vi "RemoveBus.vi"(7 "Remove All? (F)":bool, 8 "ErrorArray In":errorcluster[](array[cluster]), 10 "clFrontPanelControlRefs":T1) -> (0 "ErrorArray Out":errorcluster[](array[cluster]))   [LabVIEW 2014, in "Bus.lvlib" / "NISTBus.lvclass"]
uses:
  NISTBus.lvclass
  Framework/FrontPanel/TypeDefs/clFrontPanelControlRefs.ctl
  FGenPlugins/MyPluginBaseClass/TypeDef/PluginParams.ctl
  WfrmGenerator/WfrmPlugins/EventPluginBaseClass/TypeDefs/dblEvtSignalArray.ctl
  FGenPlugins/MyPluginBaseClass/TypeDef/CreateArbWfrmParams.ctl
  WfrmGenerator/WfrmPlugins/EventPluginBaseClass/TypeDefs/clEvtConfig.ctl
  WfrmGenerator/WfrmModule/PublicAPI/Arguments/Requests/dblEvtParams.ctl
  FGenPlugins/MyPluginBaseClass/TypeDef/ConfigArbWfrmParams.ctl
  FGenPlugins/MyPluginBaseClass/TypeDef/TriggerParams.ctl
  <userlib>/NIST/ModuleAdminLib/ModuleAdmin/ModuleAdmin.lvclass
  <vilib>/Utility/error.llb/Error Cluster From Error Code.vi
  <vilib>/ErrorRing/Error Ring.xnode
  <userlib>/NIST/NISTErrorLib/NISTErrorLib.lvlib
  FGenModule/FGenModule.lvlib
  WfrmGenerator/WfrmModule/WfrmModule.lvlib
  Framework/TestFramework.lvlib
  Bus.lvlib
  FGenPlugins/MyPluginBaseClass/NISTFGenPluginsBase.lvclass
  WfrmGenerator/WfrmPlugins/EventPluginBaseClass/BaseWfrmPlugin.lvclass
panel:
  # "When you add a control \non the front panel, add a\nreference for it in this\ntype def.  This cluster\nwill hold all of the refer-\nences to the front panel\ncontrols in order to pass\nthese control references \nto subvis."
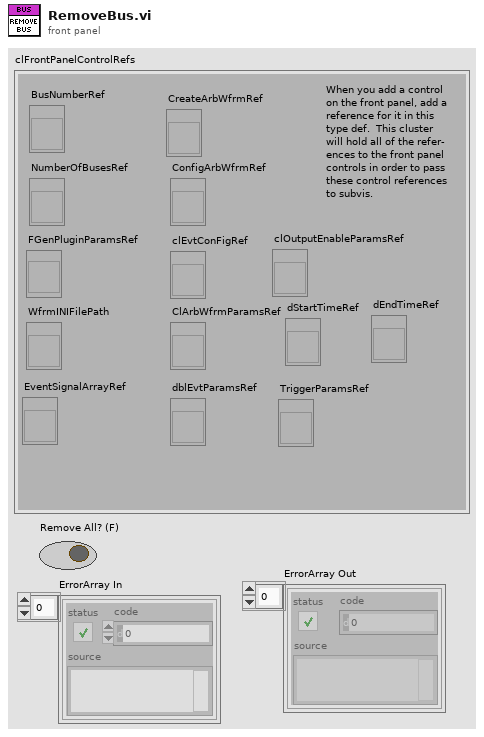
[diagram p1: front panel]
types:
  T1 = typedef "TestFramework.lvlib/clFrontPanelControlRefs.ctl" = cluster{"BusNumberRef":refnum<vi>, "NumberOfBusesRef":refnum<vi>, "FGenPluginParamsRef":refnum<vi>, "WfrmINIFilePath":refnum<vi>, "EventSignalArrayRef":refnum<vi>, "CreateArbWfrmRef":refnum<vi>, "clEvtConFigRef":refnum<vi>, "dblEvtParamsRef":refnum<vi>, "clOutputEnableParamsRef":refnum<vi>, "ConfigArbWfrmRef":refnum<vi>, "ClArbWfrmParamsRef":refnum<vi>, "dStartTimeRef":refnum<vi>, "dEndTimeRef":refnum<vi>, "TriggerParamsRef":refnum<vi>}
  T2 = typedef "TestFramework.lvlib/clFrameworkData.ctl" = cluster{"NISTBusClassInstances":refnum<class "NISTBus.lvclass">[], "NISTFGenINIFilePaths":path[], "NISTWfrmINIFilePaths":path[]}
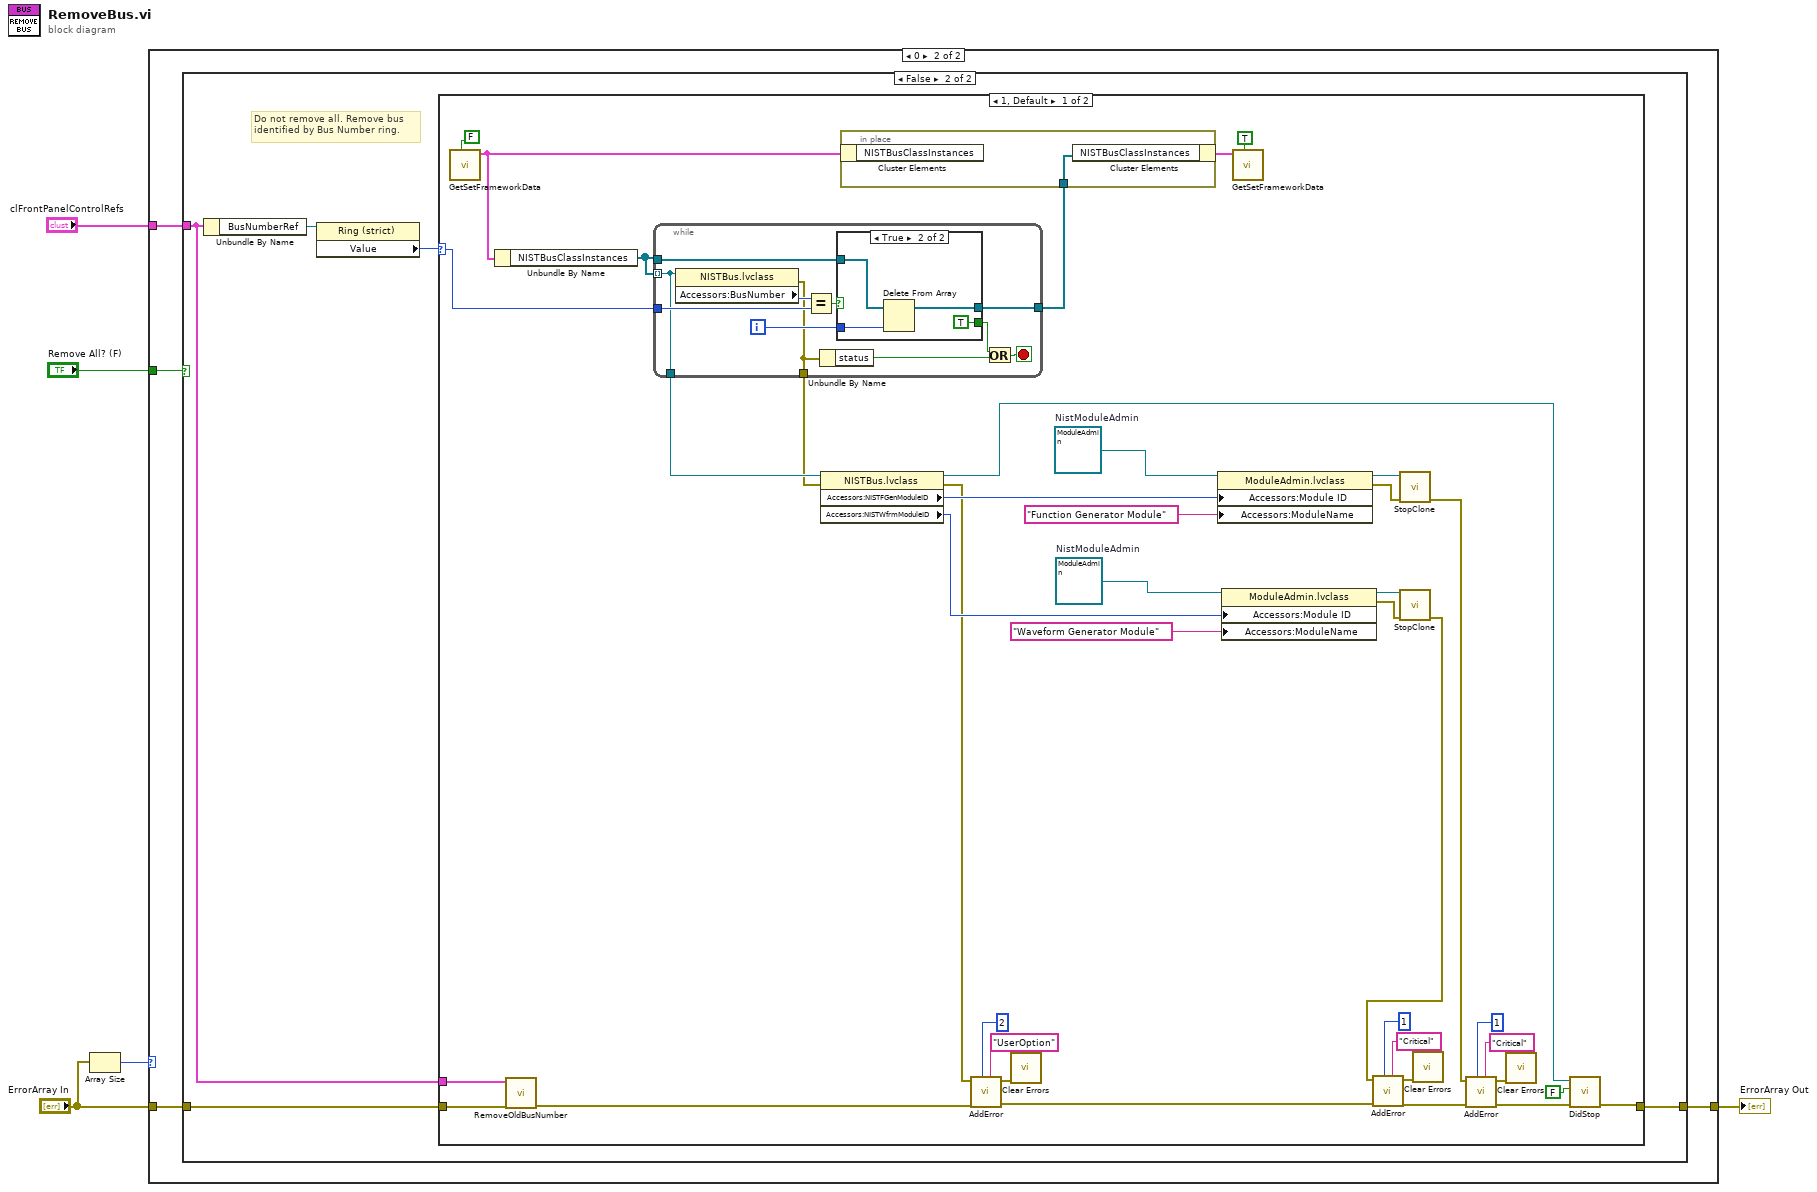
[diagram p0: block diagram]
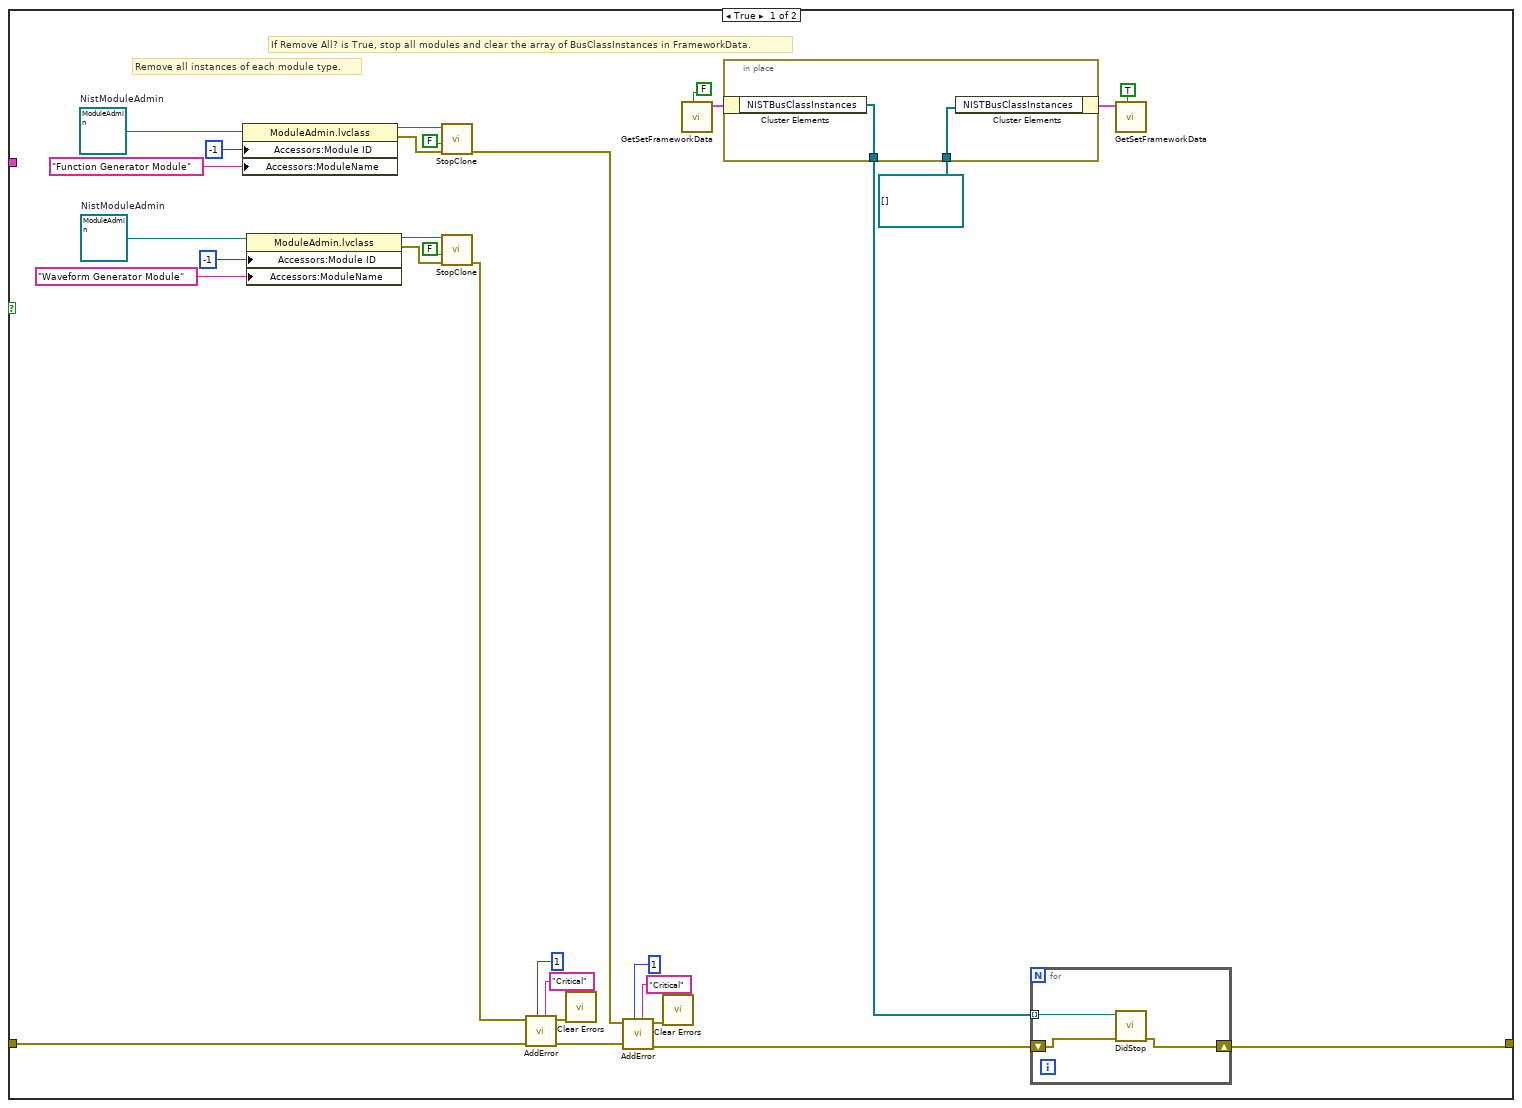
[diagram p3: hidden frame]
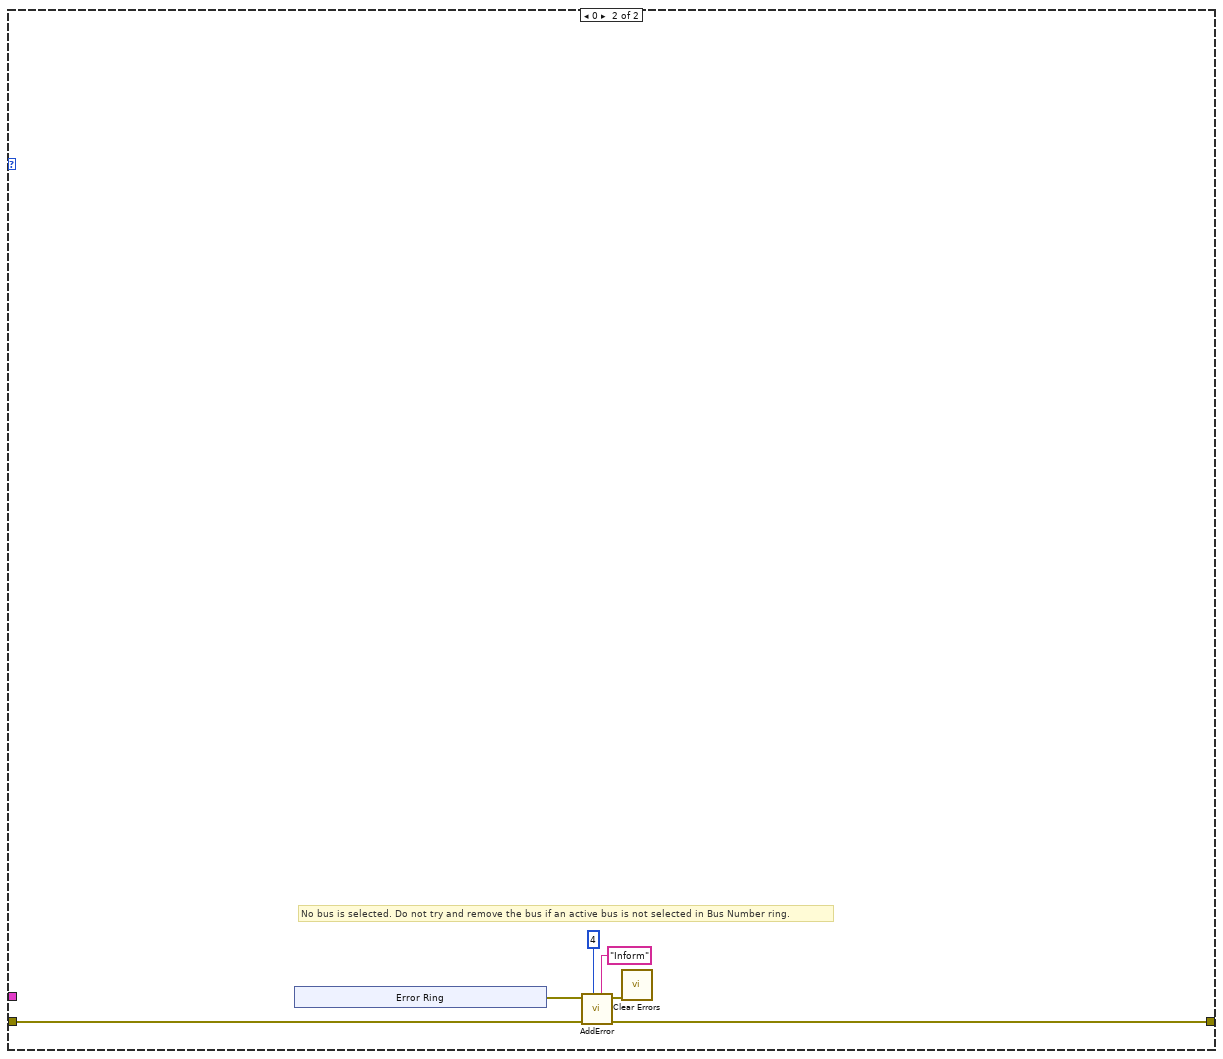
[diagram p5: hidden frame]
diagram:
  n1 = Array Size(array="ErrorArray In") -> (size(s)=w5:i32)
  n2 = case shown="0" w5 {
    tunnel: "ErrorArray In" -> [w6 w10]
    tunnel: [w6 w7] -> w3
    tunnel: "Remove All? (F)" -> [_ w9]
    tunnel: "clFrontPanelControlRefs" -> [_ w8]
    frame 1, Default {
      # "External error. Array holds error."
    }
    frame 0 {
      n3 = case shown="False" w9 {
        tunnel: w10 -> [w21 w50]
        tunnel: w8 -> [_ w47]
        tunnel: [w11 w46] -> w7
        frame True {
          w37 = refnum<class "ModuleAdmin.lvclass"> refnum  # NistModuleAdmin
          w40 = refnum<class "ModuleAdmin.lvclass"> refnum  # NistModuleAdmin
          # "Remove all instances of each module type."
          # "If Remove All? is True, stop all modules and clear the array of BusClassInstances in FrameworkData."
          n4 = property class="ModuleAdmin.lvclass"(reference=w40, "Accessors:Module ID"=-1 ("Module ID"), "Accessors:ModuleName"="Function Generator Module" ("ModuleName")) -> (reference out=w33:refnum<class "ModuleAdmin.lvclass">, error out=w32:errorcluster)  [unwired: 1 in]
          n5 = property class="ModuleAdmin.lvclass"(reference=w37, "Accessors:Module ID"=-1 ("Module ID"), "Accessors:ModuleName"="Waveform Generator Module" ("ModuleName")) -> (reference out=w31:refnum<class "ModuleAdmin.lvclass">, error out=w29:errorcluster)  [unwired: 1 in]
          n6 = call "StopClone.vi"("error in (no error)"=w32, "Wait for Module to stop?"=FALSE, "ModuleAdmin"=w33) -> ("error out"=w19:errorcluster)  [unwired: 8 in]
          n7 = call "StopClone.vi"("error in (no error)"=w29, "Wait for Module to stop?"=FALSE, "ModuleAdmin"=w31) -> ("error out"=w20:errorcluster)  [unwired: 8 in]
          n8 = call <userlib>:"AddError.vi"("Severity"="Critical" ("String"), "Priority"=u8 1, "ErrorArray"=w21, "error in (no error)"=w20) -> ("ErrorArray"=w22:errorcluster[], "error out"=w23:errorcluster)  [unwired: 6 in]
          n9 = call <vilib>:"Clear Errors.vi"("error in (no error)"=w23) -> ()  [unwired: 5 in, 2 out]
          n10 = call <userlib>:"AddError.vi"("Severity"="Critical" ("String"), "Priority"=u8 1, "ErrorArray"=w22, "error in (no error)"=w19) -> ("ErrorArray"=w12:errorcluster[], "error out"=w28:errorcluster)  [unwired: 6 in]
          n11 = call <vilib>:"Clear Errors.vi"("error in (no error)"=w28) -> ()  [unwired: 5 in, 2 out]
          n12 = call "GetSetFrameworkData.vi"("Set (F)"=FALSE) -> ("clFrameworkData Out"=w17:T2)  [unwired: 10 in]
          n13 = in-place {
            in-place-border: refnum<class "NISTBus.lvclass">[] [] ("NISTBusClassInstances") -> [w45]
            in-place-border: [w44] -> w13
            n14 = in-place-cluster #1(w17) -> ("NISTBusClassInstances"=w44:refnum<class "NISTBus.lvclass">[])
            n15 = in-place-cluster #1("NISTBusClassInstances"=w45) -> (w16:T2)
          }
          n16 = for {
            tunnel: w13 -> [w43] mode=indexing
            shift-right: [w41] -> w11
            shift-left: w12 -> [w42]
            n17 = call "DidStop.vi"("ErrorArray In"=w42, "NISTBus In"=w43) -> ("ErrorArray Out"=w41:errorcluster[])  [unwired: 8 in, 1 out]
          }
          n18 = call "GetSetFrameworkData.vi"("Set (F)"=TRUE, "clFrameworkData In"=w16) -> ()  [unwired: 9 in, 1 out]
        }
        frame False {
          # "Do not remove all. Remove bus\nidentified by Bus Number ring."
          n19 = Unbundle By Name(w47) -> ("BusNumberRef"=w49:refnum<vi>)
          n20 = property class="Ring (strict)"(reference=w49) -> ("Value"=w48:u8)  [unwired: 1 in, 2 out]
          n21 = case shown="1, Default" w48 {
            selector: w48 -> [w77 _]
            tunnel: w50 -> [w66 w113]
            tunnel: w47 -> [w67 _]
            tunnel: [w53 w112] -> w46
            frame 1, Default {
              w88 = refnum<class "ModuleAdmin.lvclass"> refnum  # NistModuleAdmin
              w90 = refnum<class "ModuleAdmin.lvclass"> refnum  # NistModuleAdmin
              n22 = call "GetSetFrameworkData.vi"("Set (F)"=FALSE) -> ("clFrameworkData Out"=w79:T2)  [unwired: 10 in]
              n23 = Unbundle By Name(w79) -> ("NISTBusClassInstances"=w78:refnum<class "NISTBus.lvclass">[])
              n24 = call "RemoveOldBusNumber.vi"("ErrorArray In"=w66, "clFrontPanelControlRefs In"=w67) -> ("ErrorArray Out"=w65:errorcluster[])  [unwired: 8 in, 1 out]
              n25 = while {
                tunnel: w77 -> [w99]
                tunnel: w78 -> [w95] mode=indexing
                tunnel: w78 -> [w98]
                tunnel: [w96] -> w76
                tunnel: [w95] -> w75
                tunnel: [w92] -> w74
                i -> [w97]
                stop <- w94 stop-if-true
                n26 = property class="NISTBus.lvclass"(reference=w95) -> (error out=w92:errorcluster, "Accessors:BusNumber"=w101:u8)  [unwired: 1 in, 1 out]
                n27 = Equal?(x=w101, y=w99) -> (x = y?=w100:bool)
                n28 = Unbundle By Name(w92) -> ("status"=w91:bool)
                n29 = case shown="True" w100 {
                  tunnel: w98 -> [w102 w106]
                  tunnel: w97 -> [_ w105]
                  tunnel: [_ TRUE] -> w93
                  tunnel: [w102 w103] -> w96
                  frame False {
                  }
                  frame True {
                    n30 = Delete From Array(array=w106, index=w105) -> (array with subset deleted=w103:refnum<class "NISTBus.lvclass">[])  [unwired: 1 in, 1 out]
                  }
                }
                n31 = Or(x=w93, y=w91) -> (x .or. y?=w94:bool)
              }
              n32 = property class="NISTBus.lvclass"(reference=w75, error in=w74) -> (reference out=w52:refnum<class "NISTBus.lvclass">, error out=w68:errorcluster, "Accessors:NISTFGenModuleID"=w73:i32, "Accessors:NISTWfrmModuleID"=w72:i32)
              n33 = in-place {
                in-place-border: w76 -> [w107]
                n34 = in-place-cluster #2(w79) -> ()  [unwired: 1 out]
                n35 = in-place-cluster #2("NISTBusClassInstances"=w107) -> (w81:T2)
              }
              n36 = call <userlib>:"AddError.vi"("Severity"="UserOption" ("String"), "Priority"=u8 2, "ErrorArray"=w65, "error in (no error)"=w68) -> ("ErrorArray"=w55:errorcluster[], "error out"=w69:errorcluster)  [unwired: 6 in]
              n37 = call <vilib>:"Clear Errors.vi"("error in (no error)"=w69) -> ()  [unwired: 5 in, 2 out]
              n38 = property class="ModuleAdmin.lvclass"(reference=w90, "Accessors:Module ID"=w73, "Accessors:ModuleName"="Function Generator Module" ("ModuleName")) -> (reference out=w86:refnum<class "ModuleAdmin.lvclass">, error out=w85:errorcluster)  [unwired: 1 in]
              n39 = property class="ModuleAdmin.lvclass"(reference=w88, "Accessors:Module ID"=w72, "Accessors:ModuleName"="Waveform Generator Module" ("ModuleName")) -> (reference out=w84:refnum<class "ModuleAdmin.lvclass">, error out=w83:errorcluster)  [unwired: 1 in]
              n40 = call "GetSetFrameworkData.vi"("Set (F)"=TRUE, "clFrameworkData In"=w81) -> ()  [unwired: 9 in, 1 out]
              n41 = call "StopClone.vi"("error in (no error)"=w85, "ModuleAdmin"=w86) -> ("error out"=w57:errorcluster)  [unwired: 9 in]
              n42 = call "StopClone.vi"("error in (no error)"=w83, "ModuleAdmin"=w84) -> ("error out"=w56:errorcluster)  [unwired: 9 in]
              n43 = call <userlib>:"AddError.vi"("Severity"="Critical" ("String"), "Priority"=u8 1, "ErrorArray"=w55, "error in (no error)"=w56) -> ("ErrorArray"=w58:errorcluster[], "error out"=w61:errorcluster)  [unwired: 6 in]
              n44 = call <vilib>:"Clear Errors.vi"("error in (no error)"=w61) -> ()  [unwired: 5 in, 2 out]
              n45 = call <userlib>:"AddError.vi"("Severity"="Critical" ("String"), "Priority"=u8 1, "ErrorArray"=w58, "error in (no error)"=w57) -> ("ErrorArray"=w54:errorcluster[], "error out"=w64:errorcluster)  [unwired: 6 in]
              n46 = call <vilib>:"Clear Errors.vi"("error in (no error)"=w64) -> ()  [unwired: 5 in, 2 out]
              n47 = call "DidStop.vi"("ErrorArray In"=w54, "Init?"=FALSE, "NISTBus In"=w52) -> ("ErrorArray Out"=w53:errorcluster[])  [unwired: 7 in, 1 out]
            }
            frame 0 {
              # "No bus is selected. Do not try and remove the bus if an active bus is not selected in Bus Number ring."
              n48 = xnode "Error Ring"() -> ("error out"=w108:errorcluster)
              n49 = call <userlib>:"AddError.vi"("Severity"="Inform" ("String"), "Priority"=u8 4, "ErrorArray"=w113, "error in (no error)"=w108) -> ("ErrorArray"=w112:errorcluster[], "error out"=w109:errorcluster)  [unwired: 6 in]
              n50 = call <vilib>:"Clear Errors.vi"("error in (no error)"=w109) -> ()  [unwired: 5 in, 2 out]
            }
          }
        }
      }
    }
  }
  "ErrorArray Out" <- w3
